vi "Open.vi"(8 "Error In":errorcluster, 11 "Sierra M100 In":refnum<visa-resource-name>) -> (0 "Error Out":errorcluster, 3 "Sierra M100 Out":refnum<visa-resource-name>)   [LabVIEW 2012, in "Sierra-M100.lvlib"]
doc: "This VI initializes communication with the mass flow controller (MFC). The serial port is set to 9600 baud rate, 8 data bits, 1 stop bit, no parity, and no flow control. Streaming mode is turned off and the receive buffer is cleared."
uses:
  Sierra-M100.lvlib
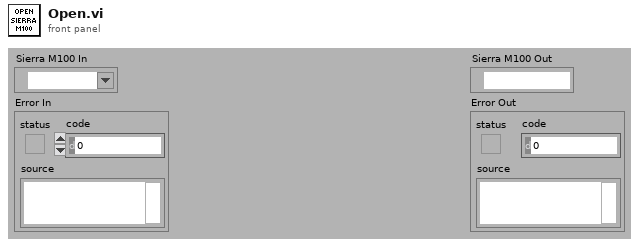
[diagram p1: front panel]
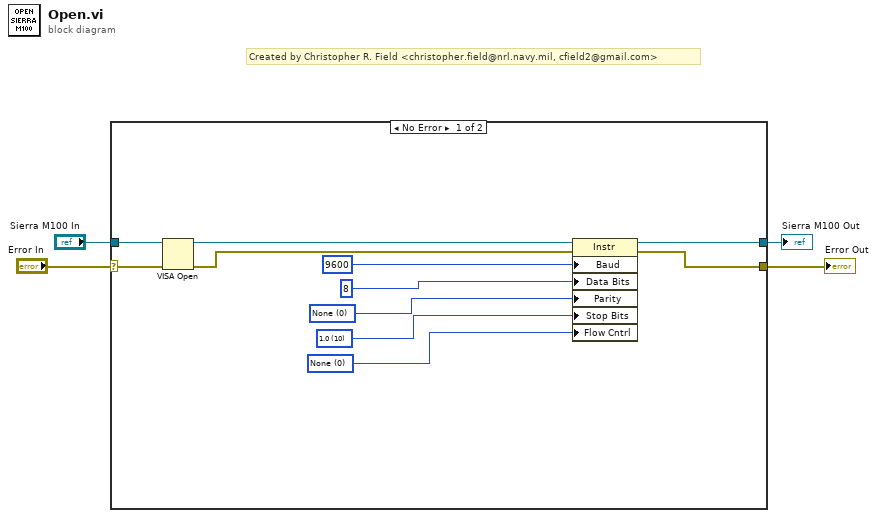
[diagram p0: block diagram]
diagram:
  # "Created by Christopher R. Field <christopher.field@nrl.navy.mil, cfield2@gmail.com>"
  n1 = case shown="No Error" "Error In" {
    selector: "Error In" -> [w5 w16]
    tunnel: "Sierra M100 In" -> [w15 w17]
    tunnel: [w7 w17] -> w3
    tunnel: [w6 w16] -> w2
    frame No Error {
      w8 = u16 0 items=["None", "XON/XOFF", "RTS/CTS", "XON/XOFF & RTS/CTS", "DTR/DSR", "XON/XOFF & DTR/DSR"] ("Serial Settings:Flow Control")
      w9 = u16 10 items=["1.0"=10, "1.5"=15, "2.0"=20] ("Serial Settings:Stop Bits")
      w10 = u16 0 items=["None", "Odd", "Even", "Mark", "Space"] ("Serial Settings:Parity")
      n2 = VISA Open(error in (no error)=w5, VISA resource name=w15) -> (VISA resource name=w14:refnum<visa-resource-name>, error out=w13:errorcluster)  [unwired: 3 in]
      n3 = property class="Instr"(reference=w14, error in=w13, "Baud"=u32 9600 ("Serial Settings:Baud Rate"), "Data Bits"=u16 8 ("Serial Settings:Data Bits"), "Parity"=w10, "Stop Bits"=w9, "Flow Cntrl"=w8) -> (reference out=w7:refnum<visa-resource-name>, error out=w6:errorcluster)
    }
    frame Error {
    }
  }
  "Sierra M100 Out" <- w3
  "Error Out" <- w2
